vi "Get_Each_channel_reference_samplingdata.vi"(0 "SPU":refnum<k24>, 1 "Ref_monitordata_struct":refnum<k24>[](array[refnum]), 2 "TSL":refnum<k24>, 3 "MPM":refnum<k24>[](array[refnum]), 4 "ChannelNumber":i32, 5 "错误输入（无错误）":errorcluster, 6 "STSProcess.PDLSTS":refnum<k24>, 7 "SweepCount":i32, 10 "Refdata_struct":refnum<k24>[](array[refnum]), 11 "SlotNumber":i32, 12 "SOP":i32, 13 "MPMNumber":i32) -> (15 "PDLSTS out":refnum<k24>, 19 "error out":errorcluster)   [LabVIEW 2017]
doc: "Get logging reference data & add in"
uses:
  D:/test/PDLSTS/LV_PDL LvVer17.0/LV_PDL_x86/DLL/STSProcess.dll
  DLL/STSProcess.dll
  D:/test/PDLSTS/LV_PDL LvVer17.0/LV_PDL_x86/DLL/InstrumentDLL.dll
  DLL/InstrumentDLL.dll
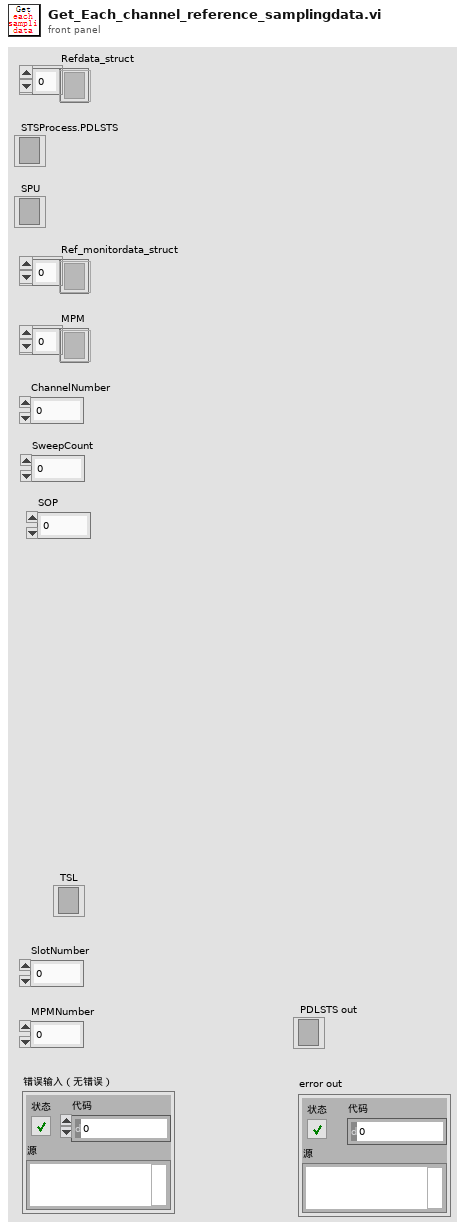
[diagram p1: front panel]
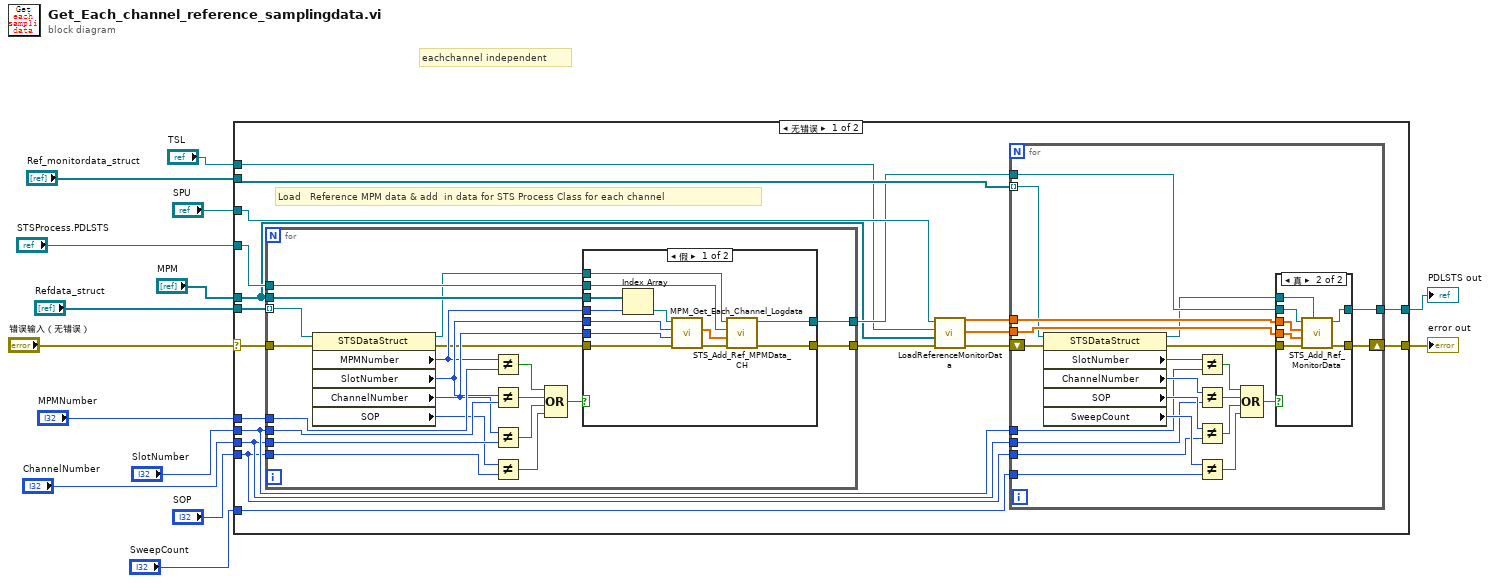
[diagram p0: block diagram]
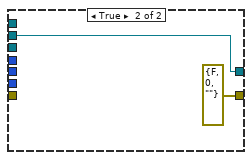
[diagram p3: hidden frame]
diagram:
  # "eachchannel independent"
  n1 = case shown="无错误" "错误输入（无错误）" {
    selector: "错误输入（无错误）" -> [w24 w101]
    tunnel: "STSProcess.PDLSTS" -> [w22 w100]
    tunnel: "Ref_monitordata_struct" -> [w30 _]
    tunnel: "SPU" -> [w29 _]
    tunnel: "MPM" -> [w15 _]
    tunnel: "ChannelNumber" -> [w19 _]
    tunnel: "SlotNumber" -> [w20 _]
    tunnel: "MPMNumber" -> [w27 _]
    tunnel: "Refdata_struct" -> [w26 _]
    tunnel: [w25 w101] -> w6
    tunnel: [w23 w100] -> w4
    tunnel: "SOP" -> [w18 _]
    tunnel: "SweepCount" -> [w17 _]
    tunnel: "TSL" -> [w16 _]
    frame No Error {
      # "Load　Reference MPM data & add  in data for STS Process Class for each channel"
      n2 = for {
        tunnel: w26 -> [w73] mode=indexing
        tunnel: w27 -> [w85]
        tunnel: w20 -> [w84]
        tunnel: w19 -> [w83]
        tunnel: w15 -> [w76]
        tunnel: w22 -> [w74]
        tunnel: [w72] -> w28
        tunnel: w24 -> [w70]
        tunnel: [w68] -> w21
        tunnel: w18 -> [w66]
        n3 = property on="属性节点" class="STSDataStruct"(reference=w73, error in=w70) -> (reference out=w69:refnum<k24>, error out=w71:errorcluster, "MPMNumber"=w75:i32, "SlotNumber"=w78:i32, "ChannelNumber"=w77:i32, "SOP"=w67:i32)
        n4 = Not Equal?(x=w75, y=w85) -> (x != y?=w82:bool)
        n5 = Not Equal?(x=w78, y=w84) -> (x != y?=w81:bool)
        n6 = Not Equal?(x=w77, y=w83) -> (x != y?=w80:bool)
        n7 = Not Equal?(x=w67, y=w66) -> (x != y?=w65:bool)
        n8 = Compound Arithmetic op=OR ("复合运算")(w82, w81, w80, w65) -> (w79:bool)
        n9 = case shown="假" w79 {
          tunnel: w78 -> [w97 _]
          tunnel: w77 -> [w96 _]
          tunnel: w76 -> [w95 _]
          tunnel: w75 -> [w93 _]
          tunnel: w74 -> [w92 w98]
          tunnel: w69 -> [w91 _]
          tunnel: [w88 errorcluster {"status"=FALSE, "code"=0, "source"=""} ("错误输出")] -> w72
          tunnel: w71 -> [w87 _]
          tunnel: [w86 w98] -> w68
          frame False {
            n10 = Index Array(array=w95, index=w93) -> (element=w94:refnum<k24>)
            n11 = call "MPM_Get_Each_Channel_Logdata.vi"("error in (no error)"=w87, "channelNumber"=w96, "moduleNumber"=w97, ".NET Reference in"=w94) -> ("error out"=w89:errorcluster, "data out"=w90:sgl[])  [unwired: 5 in, 1 out]
            n12 = call "STS_Add_Ref_MPMData_CH.vi"("错误输入（无错误）"=w89, "data"=w90, "STSProcess.PDSTS"=w92, "Setting"=w91) -> ("错误输出"=w88:errorcluster, "PDLSTS"=w86:refnum<k24>)  [unwired: 6 in]
          }
          frame True {
          }
        }
      }
      n13 = call "LoadReferenceMonitorData.vi"("错误输入（无错误）"=w28, "MPM"=w15, "TSL"=w16, "SPU"=w29) -> ("错误输出"=w31:errorcluster, "monitor"=w33:sgl[], "trigger"=w32:sgl[])  [unwired: 5 in]
      n14 = for {
        tunnel: w30 -> [w50] mode=indexing
        tunnel: w21 -> [w55]
        tunnel: w32 -> [w54]
        tunnel: w33 -> [w53]
        shift-right: [w52] -> w25
        shift-left: w31 -> [w48]
        tunnel: [w51] -> w23
        tunnel: w20 -> [w37]
        tunnel: w19 -> [w36]
        tunnel: w18 -> [w35]
        tunnel: w17 -> [w34]
        n15 = property class="STSDataStruct"(reference=w50, error in=w48) -> (reference out=w49:refnum<k24>, error out=w47:errorcluster, "SlotNumber"=w41:i32, "ChannelNumber"=w40:i32, "SOP"=w39:i32, "SweepCount"=w38:i32)
        n16 = Not Equal?(x=w41, y=w37) -> (x != y?=w46:bool)
        n17 = Not Equal?(x=w40, y=w36) -> (x != y?=w45:bool)
        n18 = Not Equal?(x=w39, y=w35) -> (x != y?=w44:bool)
        n19 = Not Equal?(x=w38, y=w34) -> (x != y?=w43:bool)
        n20 = Compound Arithmetic op=OR ("复合运算")(w46, w45, w44, w43) -> (w42:bool)
        n21 = case shown="真" w42 {
          tunnel: w55 -> [w57 w64]
          tunnel: w49 -> [_ w63]
          tunnel: w54 -> [_ w62]
          tunnel: w53 -> [_ w61]
          tunnel: w47 -> [w56 w60]
          tunnel: [w56 w59] -> w52
          tunnel: [w57 w58] -> w51
          frame False {
          }
          frame True {
            n22 = call "STS_Add_Ref_MonitorData.vi"("setting"=w63, "错误输入（无错误）"=w60, "monitorData"=w61, "triggerIndex"=w62, "STSProcess.PDLSTS"=w64) -> ("错误输出"=w59:errorcluster, "PDLSTS out"=w58:refnum<k24>)  [unwired: 5 in]
          }
        }
      }
    }
    frame Error {
    }
  }
  "error out" <- w6
  "PDLSTS out" <- w4
